vi "Set Name.vi"(8 "error in (no error)":errorcluster, 10 "Name":string, 11 "Person in":refnum<class "Person.lvclass">) -> (0 "error out":errorcluster, 3 "Person out":refnum<class "Person.lvclass">)   [LabVIEW 2023, in "Person.lvlib" / "Person.lvclass"]
doc: "Accessor method to set the Person's name."
uses:
  Person.lvclass
  Person.lvclass/Person.ctl
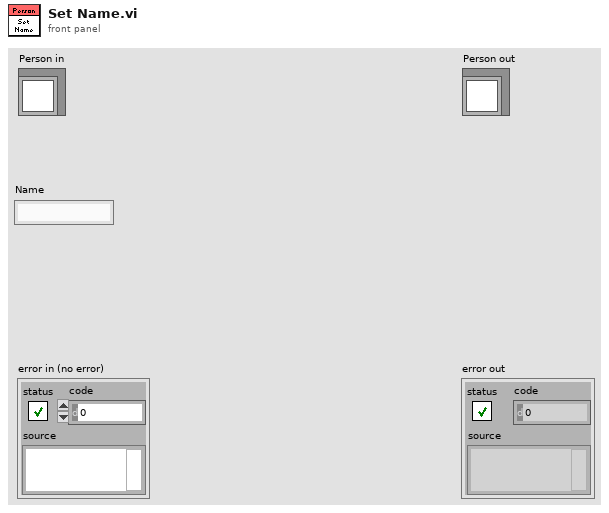
[diagram p1: front panel]
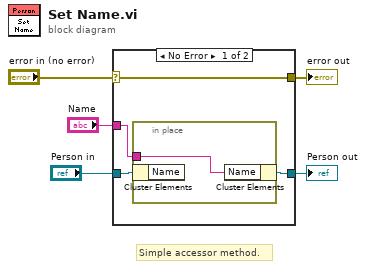
[diagram p0: block diagram]
diagram:
  # "Simple accessor method."
  n1 = case shown="No Error" "error in (no error)" {
    selector: "error in (no error)" -> [w9 w12]
    tunnel: [w9 w12] -> w4
    tunnel: [w6 w11] -> w2
    tunnel: "Person in" -> [w8 w11]
    tunnel: "Name" -> [w7 _]
    frame No Error {
      n2 = in-place "In Place Element Structure" {
        in-place-border: w7 -> [w10]
        n3 = in-place-cluster #1 ("Unbundle / Bundle Elements")(w8) -> ()  [unwired: 1 out]
        n4 = in-place-cluster #1 ("Unbundle / Bundle Elements")("Name"=w10) -> (w6:refnum<class "Person.lvclass">)
      }
    }
    frame Error {
    }
  }
  "error out" <- w4
  "Person out" <- w2
